vi "Read GD Private GV.vi"() -> ()   [LabVIEW 2026, in "TALOS.lvlib"]
uses:
  TALOS.lvlib
panel:
  out "Boolean":bool
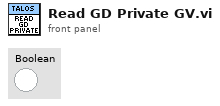
[diagram p1: front panel]
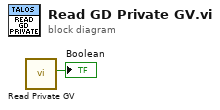
[diagram p0: block diagram]
diagram:
  n1 = call "Read Private GV.vi"() -> ("Boolean"=→"Boolean":bool)  [unwired: 11 in]
